vi "CLusterClasseEleve.vi"() -> ()   [LabVIEW 2017]
panel:
  in  "stop":bool
  out "Array 2":T1(array[cluster])
  in  "Array":T1(array[cluster])
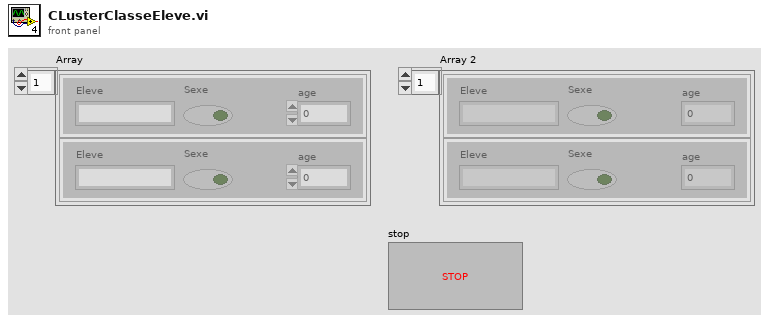
[diagram p1: front panel]
types:
  T1 = cluster{"Eleve":string, "Sexe":bool, "age":dbl}[]
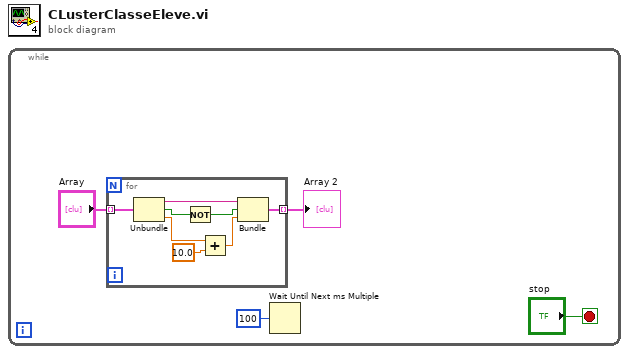
[diagram p0: block diagram]
diagram:
  n1 = while {
    stop <- "stop" stop-if-true
    n2 = for {
      tunnel: "Array" -> [w10] mode=indexing
      tunnel: [w11] -> w4 mode=indexing
      n3 = Unbundle(w10) -> ("Eleve"=w9:string, "Sexe"=w8:bool, "age"=w6:dbl)
      n4 = Not(x=w8) -> (.not. x?=w7:bool)
      n5 = Add(x=w6, y=10.0 ("x")) -> (x+y=w5:dbl)
      n6 = Bundle("Eleve"=w9, w7, w5) -> (w11:cluster{"Eleve":string, bool, dbl})  [unwired: 1 in]
    }
    "Array 2" <- w4
    n7 = Wait Until Next ms Multiple(millisecond multiple=u32 100) -> ()  [unwired: 1 out]
  }
